vi "Credito update.vi"(8 "error in (no error)":errorcluster, 10 "Credito":i32, 11 "Dinero in":refnum<class "Dinero.lvclass">) -> (0 "error out":errorcluster, 3 "Dinero out":refnum<class "Dinero.lvclass">)   [LabVIEW 2021, in "Dinero.lvlib" / "Dinero.lvclass"]
uses:
  Dinero.lvclass
  Dinero.lvclass/Dinero.ctl
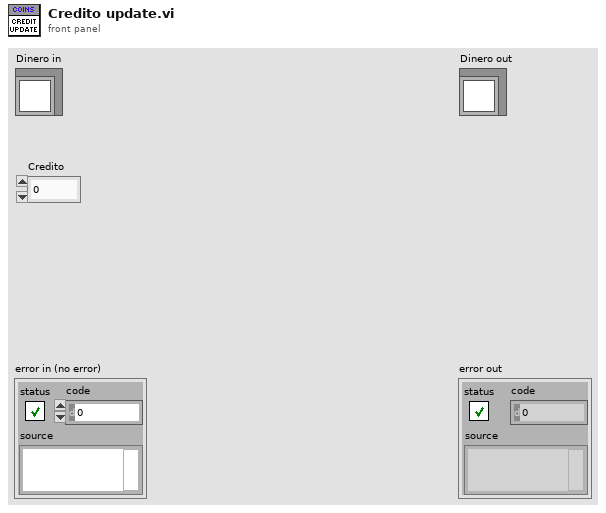
[diagram p1: front panel]
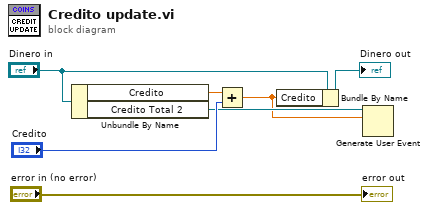
[diagram p0: block diagram]
diagram:
  n1 = Unbundle By Name("Dinero in") -> ("Credito"=w5:dbl, "Credito Total 2"=w2:refnum<user-event>)
  n2 = Add(x=w5, y="Credito") -> (x+y=w1:dbl)
  n3 = Bundle By Name(cluster="Dinero in", "Credito"=w1) -> (→"Dinero out":refnum<class "Dinero.lvclass">)
  n4 = Generate User Event(user event=w2, event data cluster=w1) -> ()  [unwired: 2 in, 2 out]
  "error out" <- "error in (no error)"
